vi "stop zeromq vi.vi"(8 "error in (no error)":errorcluster, 11 "Server in":refnum<class "Server.lvclass">) -> (0 "error out":errorcluster, 3 "Server out":refnum<class "Server.lvclass">)   [LabVIEW 2018, in "Server.lvclass"]
uses:
  Server.lvclass
  Server.lvclass/Server.ctl
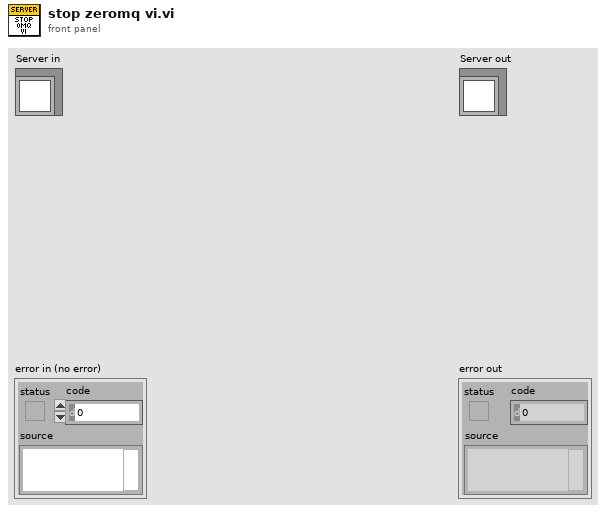
[diagram p1: front panel]
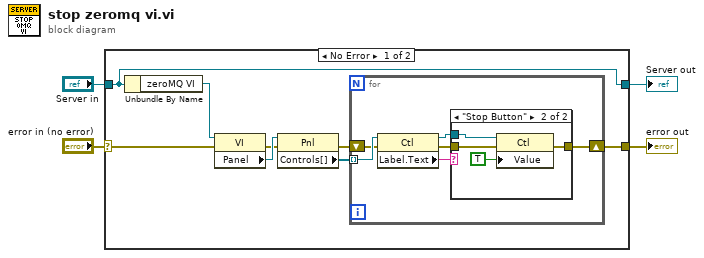
[diagram p0: block diagram]
diagram:
  n1 = case shown="No Error" "error in (no error)" {
    selector: "error in (no error)" -> [w8 w25]
    tunnel: [w5 w25] -> w3
    tunnel: [w12 w24] -> w1
    tunnel: "Server in" -> [w12 w24]
    frame No Error {
      n2 = Unbundle By Name(w12) -> ("zeroMQ VI"=w11:refnum<vi>)
      n3 = property class="VI"(reference=w11, error in=w8) -> (error out=w7:errorcluster, "Panel"=w10:refnum<vi>)  [unwired: 1 out]
      n4 = property class="Pnl"(reference=w10, error in=w7) -> (error out=w6:errorcluster, "Controls[]"=w9:refnum<vi>[])  [unwired: 1 out]
      n5 = for {
        tunnel: w9 -> [w18] mode=indexing
        shift-right: [w13] -> w5
        shift-left: w6 -> [w15]
        n6 = property class="Ctl"(reference=w18, error in=w15) -> (reference out=w16:refnum<vi>, error out=w14:errorcluster, "Label.Text"=w17:string)
        n7 = case shown="\"Stop Button\"" w17 {
          tunnel: w16 -> [_ w23]
          tunnel: w14 -> [w19 w21]
          tunnel: [w19 w20] -> w13
          frame "False", Default {
          }
          frame "Stop Button" {
            n8 = property class="Ctl"(reference=w23, error in=w21, "Value"=TRUE) -> (error out=w20:errorcluster)  [unwired: 1 out]
          }
        }
      }
    }
    frame Error {
    }
  }
  "error out" <- w3
  "Server out" <- w1
